vi "state time lookup BAP4B.vi"(7 "system state in":T1) -> (8 "system state out":T1)   [LabVIEW 2014]
doc: "This subvi looks up the light state time for the intersection state machine from an internal database. A time of -1 ms indicates no time limit.\n\nPaul K Dixon\nP350\nCSUSB Physics"
uses:
  typedefs/system state cluster.ctl
  typedefs/state enum.ctl
  typedefs/state time cluster.ctl
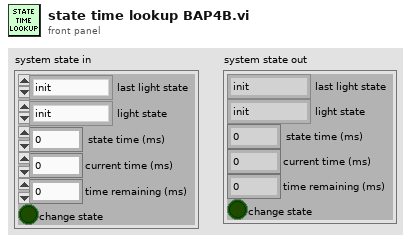
[diagram p1: front panel]
types:
  T1 = typedef "system state cluster.ctl" = cluster{"last light state":T2, "light state":T2, "state time (ms)":i32, "current time (ms)":i32, "time remaining (ms)":i32, "change state":bool}
  T2 = typedef "state enum.ctl" = enum16{"init", "idle", "left turn E", "go EW", "caution EW", "left turn W", "left turn N", "go NS", "caution NS", "left turn S", "blink on", "blink off", "all on test", "exit"}
  T3 = typedef "state time cluster.ctl" = cluster{"light state":T2, "state time (ms)":i32}
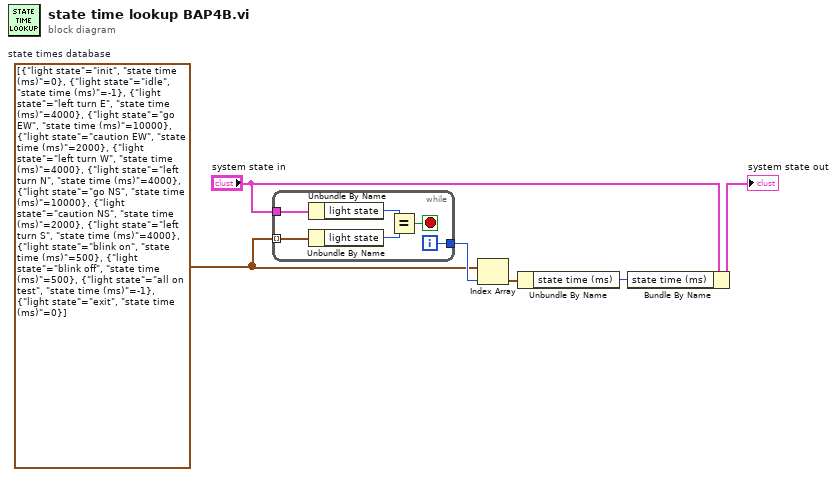
[diagram p0: block diagram]
diagram:
  w5 = T3[] [{"light state"=enum."init", "state time (ms)"=0}, {"light state"=enum."idle", "state time (ms)"=-1}, {"light state"=enum."left turn E", "state time (ms)"=4000}, {"light state"=enum."go EW", "state time (ms)"=10000}, {"light state"=enum."caution EW", "state time (ms)"=2000}, {"light state"=enum."left turn W", "state time (ms)"=4000}, {"light state"=enum."left turn N", "state time (ms)"=4000}, {"light state"=enum."go NS", "state time (ms)"=10000}, {"light state"=enum."caution NS", "state time (ms)"=2000}, {"light state"=enum."left turn S", "state time (ms)"=4000}, {"light state"=enum."blink on", "state time (ms)"=500}, {"light state"=enum."blink off", "state time (ms)"=500}, {"light state"=enum."all on test", "state time (ms)"=-1}, {"light state"=enum."exit", "state time (ms)"=0}]  # state times database
  n1 = while {
    tunnel: w5 -> [w12] mode=indexing
    tunnel: "system state in" -> [w10]
    tunnel: [w7] -> w6
    i -> [w7]
    stop <- w8 stop-if-true
    n2 = Unbundle By Name(w10) -> ("light state"=w9:T2)
    n3 = Unbundle By Name(w12) -> ("light state"=w11:T2)
    n4 = Equal?(x=w9, y=w11) -> (x = y?=w8:bool)
  }
  n5 = Index Array(array=w5, index=w6) -> (element=w4:T3)
  n6 = Unbundle By Name(w4) -> ("state time (ms)"=w2:i32)
  n7 = Bundle By Name(cluster="system state in", "state time (ms)"=w2) -> (→"system state out":T1)
